vi "Save Logging Settings to File.vi"(0 "Logging Settings":T1={"Logging Interval [s]"=1.0, "Use Lowpass Filter"=TRUE, "Tf [s]"=5.0, "Logging Data to File"=TRUE, "Log Folder"=path "c:/Temp/Data.lvm", "Logging Data to Cloud Service"=FALSE, "Data Cloud Service Url"="http://127.0.0.1:8001/DataWS", "Use Random Data"=TRUE}, 11 "Error In":errorcluster) -> (15 "Error Out":errorcluster)   [LabVIEW 2019]
uses:
  Controls/Logging Settings.ctl
  <vilib>/Utility/config.llb/Write Key (Double).vi
  <vilib>/Utility/config.llb/Write Key (Boolean).vi
  <vilib>/Utility/config.llb/Write Key (Path).vi
  <vilib>/Utility/config.llb/Write Key (String).vi
  <vilib>/Utility/config.llb/NI_LVConfig.lvlib
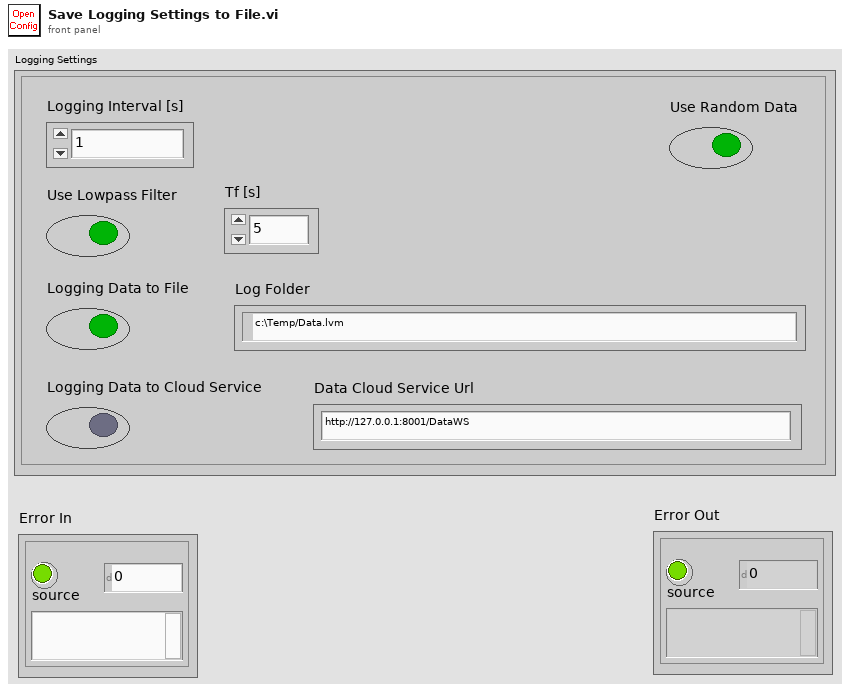
[diagram p1: front panel]
types:
  T1 = typedef "Logging Settings.ctl" = cluster{"Logging Interval [s]":dbl, "Use Lowpass Filter":bool, "Tf [s]":dbl, "Logging Data to File":bool, "Log Folder":path, "Logging Data to Cloud Service":bool, "Data Cloud Service Url":string, "Use Random Data":bool}
  T2 = typedef "NI_LVConfig.lvlib/Config Data RefNum.ctl" = refnum<k1>
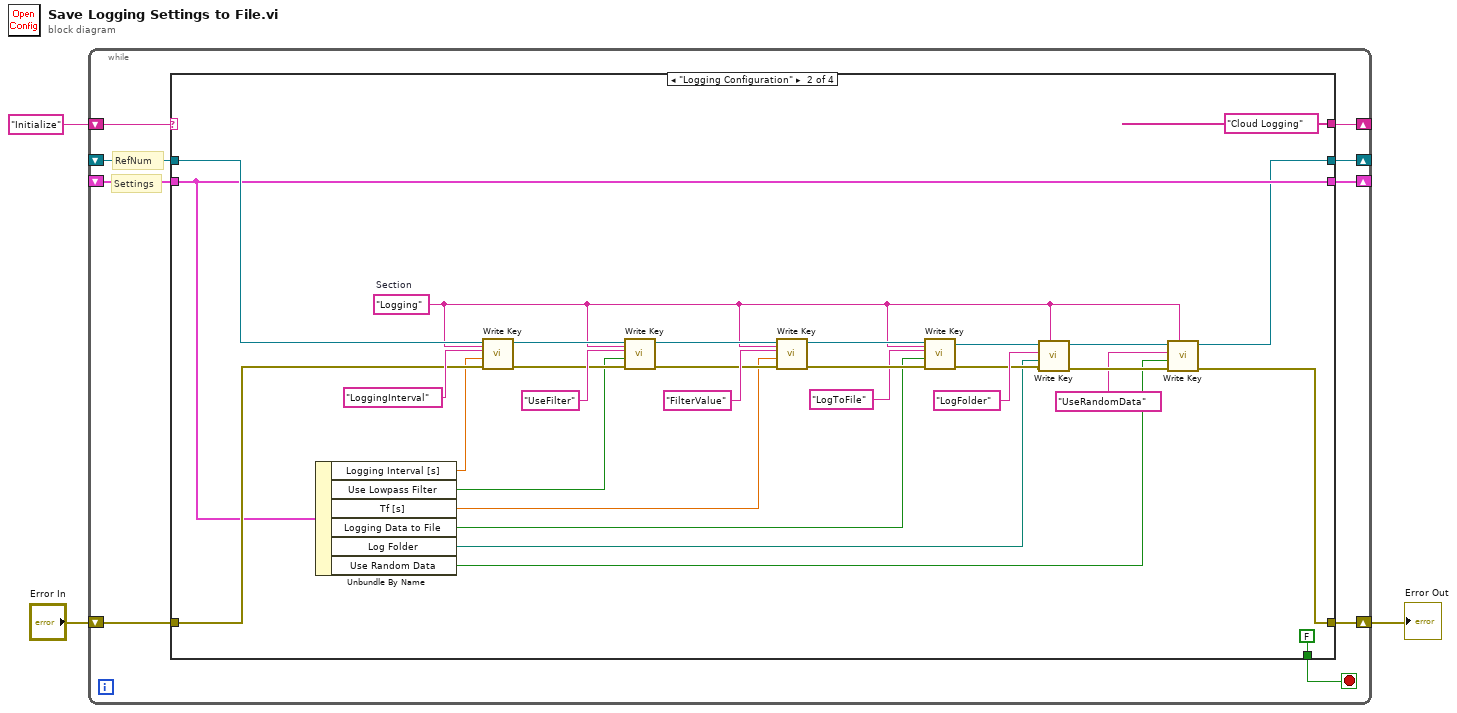
[diagram p0: block diagram]
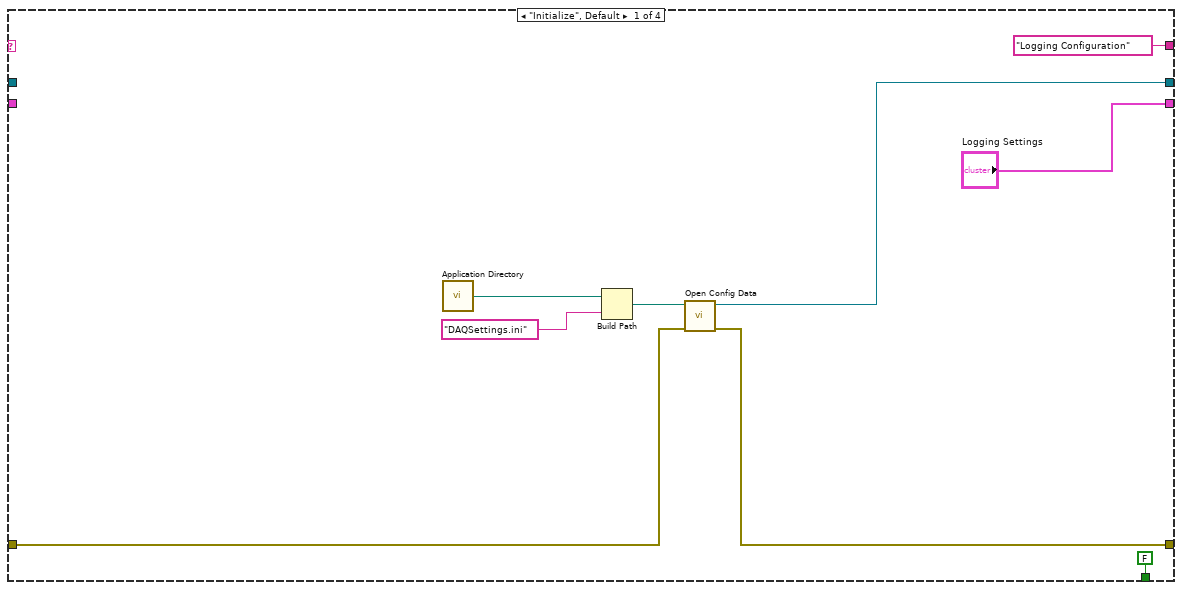
[diagram p2: hidden frame]
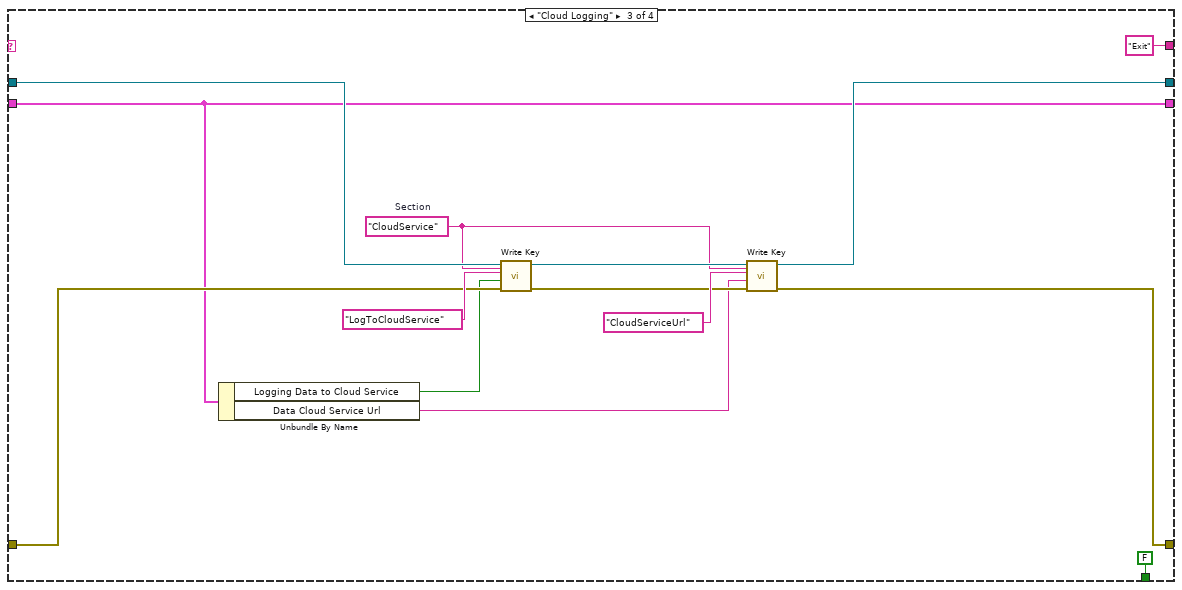
[diagram p3: hidden frame]
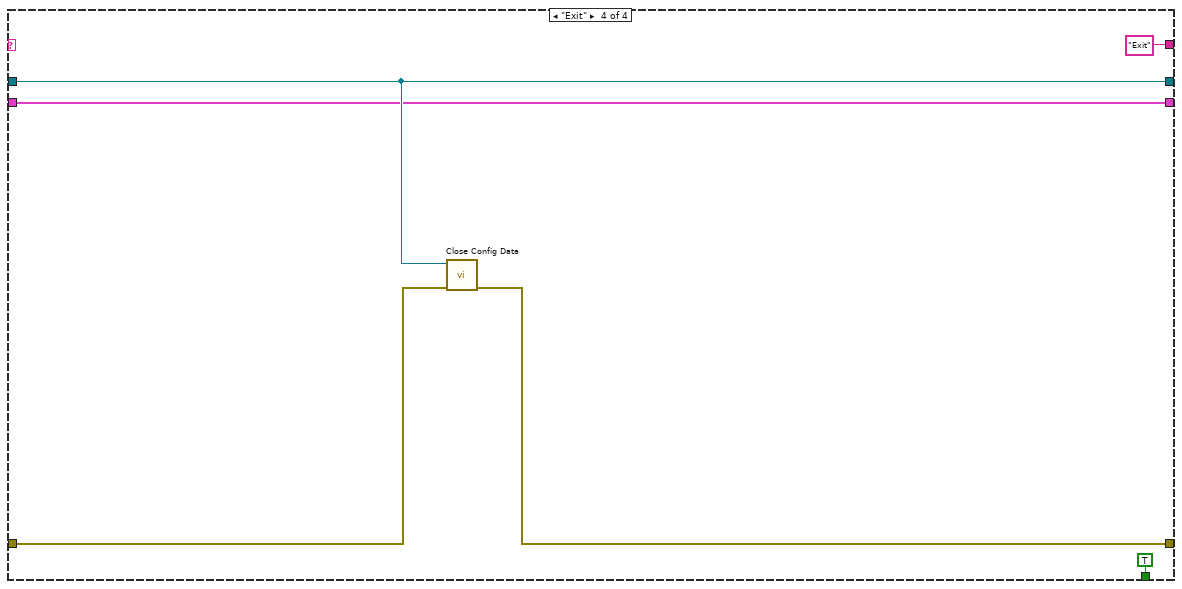
[diagram p4: hidden frame]
diagram:
  n1 = while {
    shift-right: [w7] -> _
    shift-left: "Initialize" ("key") -> [w12]
    shift-right: [w8] -> _
    shift-left: _ -> [w11]
    shift-right: [w9] -> w1
    shift-left: "Error In" -> [w10]
    shift-right: [w4] -> _
    shift-left: _ -> [w5]
    stop <- w6 stop-if-true
    # "Settings"
    # "RefNum"
    n2 = case shown="\"Logging Configuration\"" w12 {
      tunnel: w11 -> [_ w47 w61 w69]
      tunnel: w10 -> [w21 w46 w60 w71]
      tunnel: [w20 w26 w55 w70] -> w9
      tunnel: [w19 w23 w56 w69] -> w8
      tunnel: ["Logging Configuration" ("key") "Cloud Logging" ("key") "Exit" ("key") "Exit" ("key")] -> w7
      tunnel: [FALSE FALSE FALSE TRUE] -> w6
      tunnel: w5 -> [_ w29 w52 w66]
      tunnel: ["Logging Settings" w29 w52 w66] -> w4
      frame "Initialize", Default {
        n3 = call <vilib>:"Application Directory.vi"() -> ("Application Directory"=w16:path)
        n4 = Build Path(base path=w16, name or relative path="DAQSettings.ini") -> (appended path=w14:path)
        n5 = call <vilib>:"Open Config Data.vi"("error in (no error)"=w21, "configuration file path"=w14) -> ("error out"=w20:errorcluster, "refnum"=w19:T2)  [unwired: 7 in, 1 out]
      }
      frame "Logging Configuration" {
        w22 = "Logging"  # Section
        n6 = Unbundle By Name(w29) -> ("Logging Interval [s]"=w34:dbl, "Use Lowpass Filter"=w33:bool, "Tf [s]"=w32:dbl, "Logging Data to File"=w31:bool, "Log Folder"=w30:path, "Use Random Data"=w25:bool)
        n7 = call-poly <vilib>:"Write Key.vi"("section"=w22, "error in (no error)"=w46, "value"=w34, "key"="LoggingInterval", "refnum"=w47) -> ("error out"=w50:errorcluster, "refnum out"=w49:T2)  [unwired: 4 in, 1 out]
        n8 = call-poly <vilib>:"Write Key.vi"("section"=w22, "error in (no error)"=w50, "value"=w33, "key"="UseFilter", "refnum"=w49) -> ("error out"=w41:errorcluster, "refnum out"=w42:T2)  [unwired: 4 in, 1 out]
        n9 = call-poly <vilib>:"Write Key.vi"("section"=w22, "error in (no error)"=w41, "value"=w32, "key"="FilterValue", "refnum"=w42) -> ("error out"=w39:errorcluster, "refnum out"=w40:T2)  [unwired: 4 in, 1 out]
        n10 = call-poly <vilib>:"Write Key.vi"("section"=w22, "error in (no error)"=w39, "value"=w31, "key"="LogToFile", "refnum"=w40) -> ("error out"=w36:errorcluster, "refnum out"=w37:T2)  [unwired: 4 in, 1 out]
        n11 = call-poly <vilib>:"Write Key.vi"("section"=w22, "error in (no error)"=w36, "value"=w30, "key"="LogFolder", "refnum"=w37) -> ("error out"=w28:errorcluster, "refnum out"=w24:T2)  [unwired: 4 in, 1 out]
        n12 = call-poly <vilib>:"Write Key.vi"("section"=w22, "error in (no error)"=w28, "value"=w25, "key"="UseRandomData", "refnum"=w24) -> ("error out"=w26:errorcluster, "refnum out"=w23:T2)  [unwired: 4 in, 1 out]
      }
      frame "Cloud Logging" {
        w57 = "CloudService"  # Section
        n13 = Unbundle By Name(w52) -> ("Logging Data to Cloud Service"=w54:bool, "Data Cloud Service Url"=w53:string)
        n14 = call-poly <vilib>:"Write Key.vi"("section"=w57, "error in (no error)"=w60, "value"=w54, "key"="LogToCloudService", "refnum"=w61) -> ("error out"=w64:errorcluster, "refnum out"=w63:T2)  [unwired: 4 in, 1 out]
        n15 = call-poly <vilib>:"Write Key.vi"("section"=w57, "error in (no error)"=w64, "value"=w53, "key"="CloudServiceUrl", "refnum"=w63) -> ("error out"=w55:errorcluster, "refnum out"=w56:T2)  [unwired: 4 in, 1 out]
      }
      frame "Exit" {
        n16 = call <vilib>:"Close Config Data.vi"("error in (no error)"=w71, "refnum"=w69) -> ("error out"=w70:errorcluster)  [unwired: 8 in, 1 out]
      }
    }
  }
  "Error Out" <- w1
